vi "ABR-Parse Data.vi"(0 "Data":dbl[](array[numeric]), 1 "Reject OverRide":bool, 2 "Rej Thresh µV":dbl=15.0, 7 "scale factor":dbl=1.0, 9 "Acquired In":i32, 11 "error in (no error)":errorcluster, 12 "Runtime":T1) -> (3 "Finished?":bool, 4 "Any rejected?":bool, 6 "RunSum1":dbl[](array[numeric]), 8 "RunSum2":dbl[](array[numeric]), 10 "Acquired Out":i32, 14 "Ntries":i32, 15 "error out":errorcluster)   [LabVIEW 2020]
uses:
  Typedefs/ABR-Runtime Data.ctl
  epl-vi-lib/Signal Synthesis VIs/4th Generation/Classes/SignalManager/SignalManager.lvclass
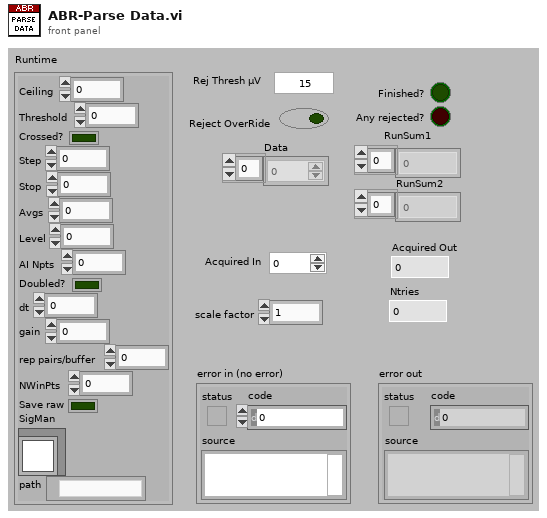
[diagram p1: front panel]
types:
  T1 = typedef "ABR-Runtime Data.ctl" = cluster{"Ceiling":dbl, "Threshold":dbl, "Crossed?":bool, "Step":dbl, "Stop":i32, "Avgs":i32, "Level":dbl, "AI Npts":i32, "Doubled?":bool, "dt":dbl, "gain":dbl, "rep pairs/buffer":i32, "NWinPts":i32, "Save raw":bool, "SigMan":refnum<class "SignalManager.lvclass">, "path":path}
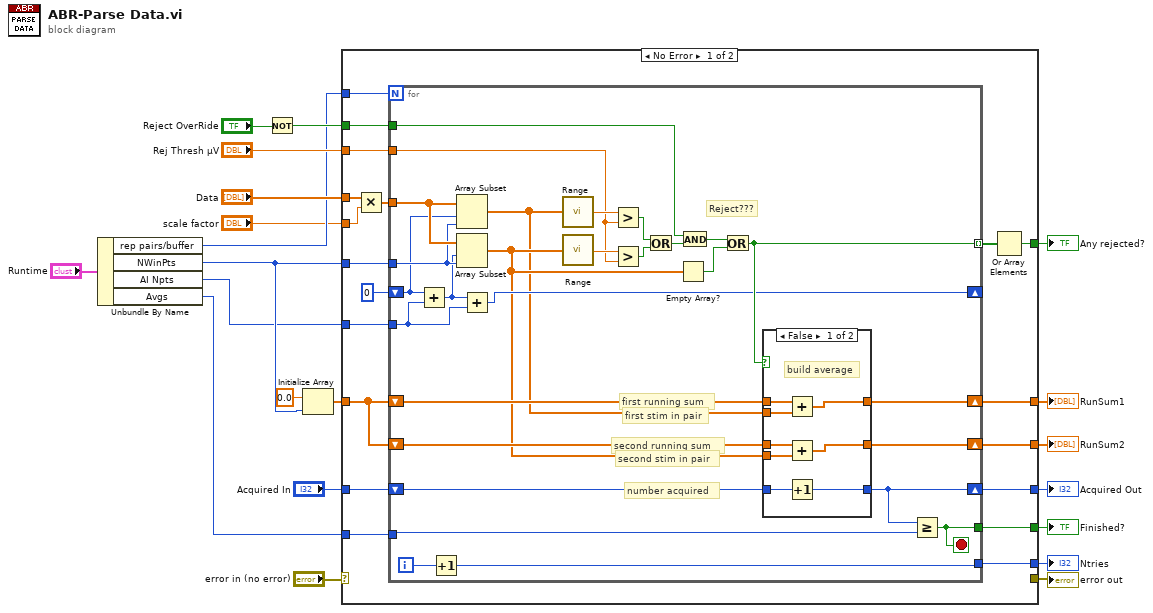
[diagram p0: block diagram]
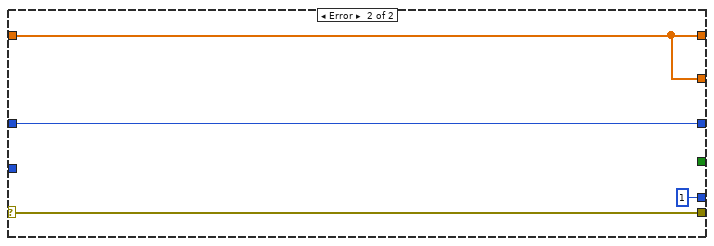
[diagram p3: hidden frame]
diagram:
  n1 = Unbundle By Name("Runtime") -> ("rep pairs/buffer"=w5:i32, "NWinPts"=w9:i32, "AI Npts"=w1:i32, "Avgs"=w8:i32)
  n2 = Not(x="Reject OverRide") -> (.not. x?=w17:bool)
  n3 = Initialize Array(0.0 ("element"), w9) -> (w13:dbl[])
  n4 = case shown="No Error" "error in (no error)" {
    selector: "error in (no error)" -> [_ w83]
    tunnel: [_ w83] -> w20
    tunnel: "Data" -> [w40 _]
    tunnel: w17 -> [w39 _]
    tunnel: "Rej Thresh µV" -> [w38 _]
    tunnel: w9 -> [w37 _]
    tunnel: w5 -> [w36 _]
    tunnel: w1 -> [w35 _]
    tunnel: [w33 _] -> w14
    tunnel: w13 -> [w32 w81]
    tunnel: [w30 w81] -> w2
    tunnel: [w29 w81] -> w3
    tunnel: [w28 w82] -> w12
    tunnel: "Acquired In" -> [w27 w82]
    tunnel: w8 -> [w26 _]
    tunnel: [w25 _] -> w7
    tunnel: [w24 1] -> w6
    tunnel: "scale factor" -> [w22 _]
    frame No Error {
      n5 = Multiply(x=w40, y=w22) -> (x*y=w23:dbl[])
      n6 = for {
        N: w36 -> [_]
        tunnel: w23 -> [w61]
        tunnel: w39 -> [w60]
        tunnel: w38 -> [w59]
        tunnel: w37 -> [w58]
        tunnel: w35 -> [w49]
        tunnel: [w57] -> w34 mode=indexing
        shift-right: [w47] -> w28
        shift-left: w27 -> [w56]
        shift-right: [w54] -> w30
        shift-left: w32 -> [w55]
        shift-right: [w53] -> w29
        shift-left: w32 -> [w52]
        shift-right: [w48] -> _
        shift-left: 0 -> [w51]
        tunnel: w26 -> [w46]
        tunnel: [w45] -> w25
        tunnel: [w43] -> w24
        i -> [w44]
        stop <- w45 stop-if-true
        # "Reject???"
        # "second running sum"
        # "first running sum"
        # "second stim in pair"
        # "first stim in pair"
        # "number acquired"
        n7 = Add(x=w51, y=w49) -> (x+y=w50:i32)
        n8 = Increment(x=w44) -> (x+1=w43:i32)
        n9 = Array Subset(array=w61, index=w51, length=w58) -> (w41:dbl[])
        n10 = Array Subset(array=w61, index=w50, length=w58) -> (w42:dbl[])
        n11 = Add(x=w50, y=w49) -> (x+y=w48:i32)
        n12 = call "Range.vi"("Array"=w41) -> ("Range"=w63:dbl)
        n13 = call "Range.vi"("Array"=w42) -> ("Range"=w62:dbl)
        n14 = Greater?(x=w63, y=w59) -> (0:w65:bool)
        n15 = Greater?(x=w62, y=w59) -> (0:w64:bool)
        n16 = Or(x=w65, y=w64) -> (x .or. y?=w66:bool)
        n17 = Empty Array?(array=w42) -> (empty?=w67:bool)
        n18 = And(x=w60, y=w66) -> (x .and. y?=w68:bool)
        n19 = Or(x=w68, y=w67) -> (x .or. y?=w57:bool)
        n20 = case shown="False" w57 {
          tunnel: w41 -> [w74 _]
          tunnel: w42 -> [w70 _]
          tunnel: w56 -> [w76 w79]
          tunnel: [w75 w79] -> w47
          tunnel: w55 -> [w73 w78]
          tunnel: [w72 w78] -> w54
          tunnel: [w71 w77] -> w53
          tunnel: w52 -> [w69 w77]
          frame False {
            # "build average"
            n21 = Add(x=w73, y=w74) -> (x+y=w72:dbl[])
            n22 = Add(x=w69, y=w70) -> (x+y=w71:dbl[])
            n23 = Increment(x=w76) -> (x+1=w75:i32)
          }
          frame True {
          }
        }
        n24 = Greater Or Equal?(x=w47, y=w46) -> (x >= y?=w45:bool)
      }
      n25 = Or Array Elements(Boolean array=w34) -> (logical OR=w33:bool)
    }
    frame Error {
    }
  }
  "error out" <- w20
  "Any rejected?" <- w14
  "RunSum1" <- w2
  "RunSum2" <- w3
  "Acquired Out" <- w12
  "Finished?" <- w7
  "Ntries" <- w6
